vi "RSZVB Set Receiver Step Attenuators.vi"(7 "Attenuation Factor (0.0)":dbl format="%^.3e", 8 "error in (no error)":errorcluster {"code" format="%.0x"}, 9 "Analyzer Port (0: Test Port 1)":i32(ring) items=["Test Port 1", "Test Port 2", "Test Port 3", "Test Port 4"], 10 "Channel (1)":i32=1, 11 "VISA session":refnum<visa-resource-name>) -> (0 "error out":errorcluster {"code" format="%.0x"}, 3 "dup VISA session":refnum<visa-resource-name>)   [LabVIEW 2011]
doc: "This VI sets an attenuation factor for the wave received at test port no. The generated wave is attenuated automatically if step attenuators are available.\n\nRemote-control command(s):\n[SENSe<Ch>:]POWer:ATTenuation ARECeiver | BRECeiver | CRECeiver | DRECeiver, <numeric_value>"
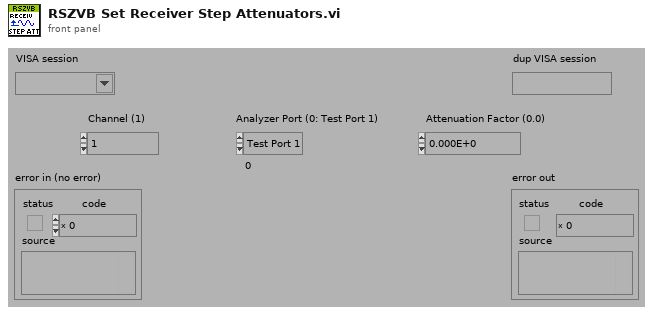
[diagram p1: front panel]
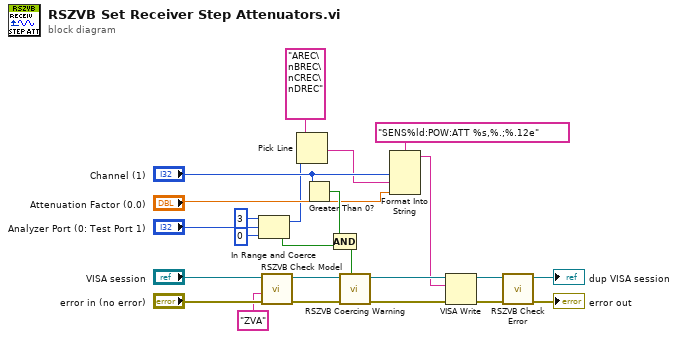
[diagram p0: block diagram]
diagram:
  n1 = In Range and Coerce(upper limit=3, x="Analyzer Port (0: Test Port 1)", lower limit=0) -> (coerced(x)=w7:i32, In Range?=w14:bool)
  n2 = call "RSZVB Check Model.vi"("error in (no error)"="error in (no error)", "Model"="ZVA" ("Options"), "VISA session"="VISA session") -> ("error out"=w5:errorcluster, "dup VISA session"=w4:refnum<visa-resource-name>)  [unwired: 7 in]
  n3 = Pick Line(multi-line string="AREC\nBREC\nCREC\nDREC", line index=w7) -> (output string=w6:string)  [unwired: 1 in]
  n4 = Greater Than 0?(x="Channel (1)") -> (x > 0?=w17:bool)
  n5 = Compound Arithmetic op=AND(w17, w14) -> (w19:bool)
  n6 = call "RSZVB Coercing Warning.vi"("In Range?"=w19, "error in (no error)"=w5, "VISA session"=w4) -> ("error out"=w22:errorcluster, "dup VISA session"=w23:refnum<visa-resource-name>)  [unwired: 7 in]
  n7 = Format Into String(format string="SENS%ld:POW:ATT %s,%.;%.12e", "Channel (1)", w6, "Attenuation Factor (0.0)") -> (resulting string=w18:string)  [unwired: 2 in, 1 out]
  n8 = VISA Write(VISA resource name=w23, write buffer=w18, error in (no error)=w22) -> (VISA resource name out=w20:refnum<visa-resource-name>, error out=w21:errorcluster)  [unwired: 1 out]
  n9 = call "RSZVB Check Error.vi"("error in (no error)"=w21, "VISA session"=w20) -> ("error out"=→"error out":errorcluster, "dup VISA session"=→"dup VISA session":refnum<visa-resource-name>)  [unwired: 8 in]
